vi "בדיקת מפל מתח בין הדקי הממסר תחת עומס 7.vi"(8 "error":errorcluster, 11 "Path for Log":path) -> (0 "error IO":errorcluster, 1 "בטווח כן/לא":bool, 2 "מפל מתח בין דקי הממסר תחת עומס":dbl, 3 "תוצאה זמנית":dbl)   [LabVIEW 2015]
uses:
  M9700 Driver/85/vi.lib/M9700 Modbus.llb/CTL Register Address.ctl
  M9700 Driver/86/vi.lib/M9700 Modbus.llb/CTL CMD Register.ctl
  <vilib>/DAQmx/write.llb/DAQmx Write (Digital Bool 1Line 1Point).vi
  <vilib>/Instr/_visa.llb/VISA Configure Serial Port (Instr).vi
  <vilib>/DAQmx/create/channels.llb/DAQmx Create Channel (DO-Digital Output).vi
  <vilib>/DAQmx/miscellaneous.llb/DAQmx Fill In Error Info.vi
panel:
  out "progress":dbl(slide) min=0.0 max=10.0 scale=0.0..10.0
  in  "stop":bool
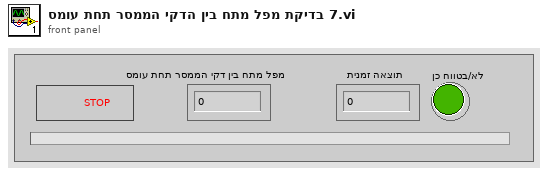
[diagram p1: front panel]
types:
  T1 = enum32{"Invalid", "Standard", "Closed", "Hidden", "Minimized", "Maximized"}
  T2 = typedef "CTL CMD Register.ctl" = u8
  T3 = typedef "CTL Register Address.ctl" = u16
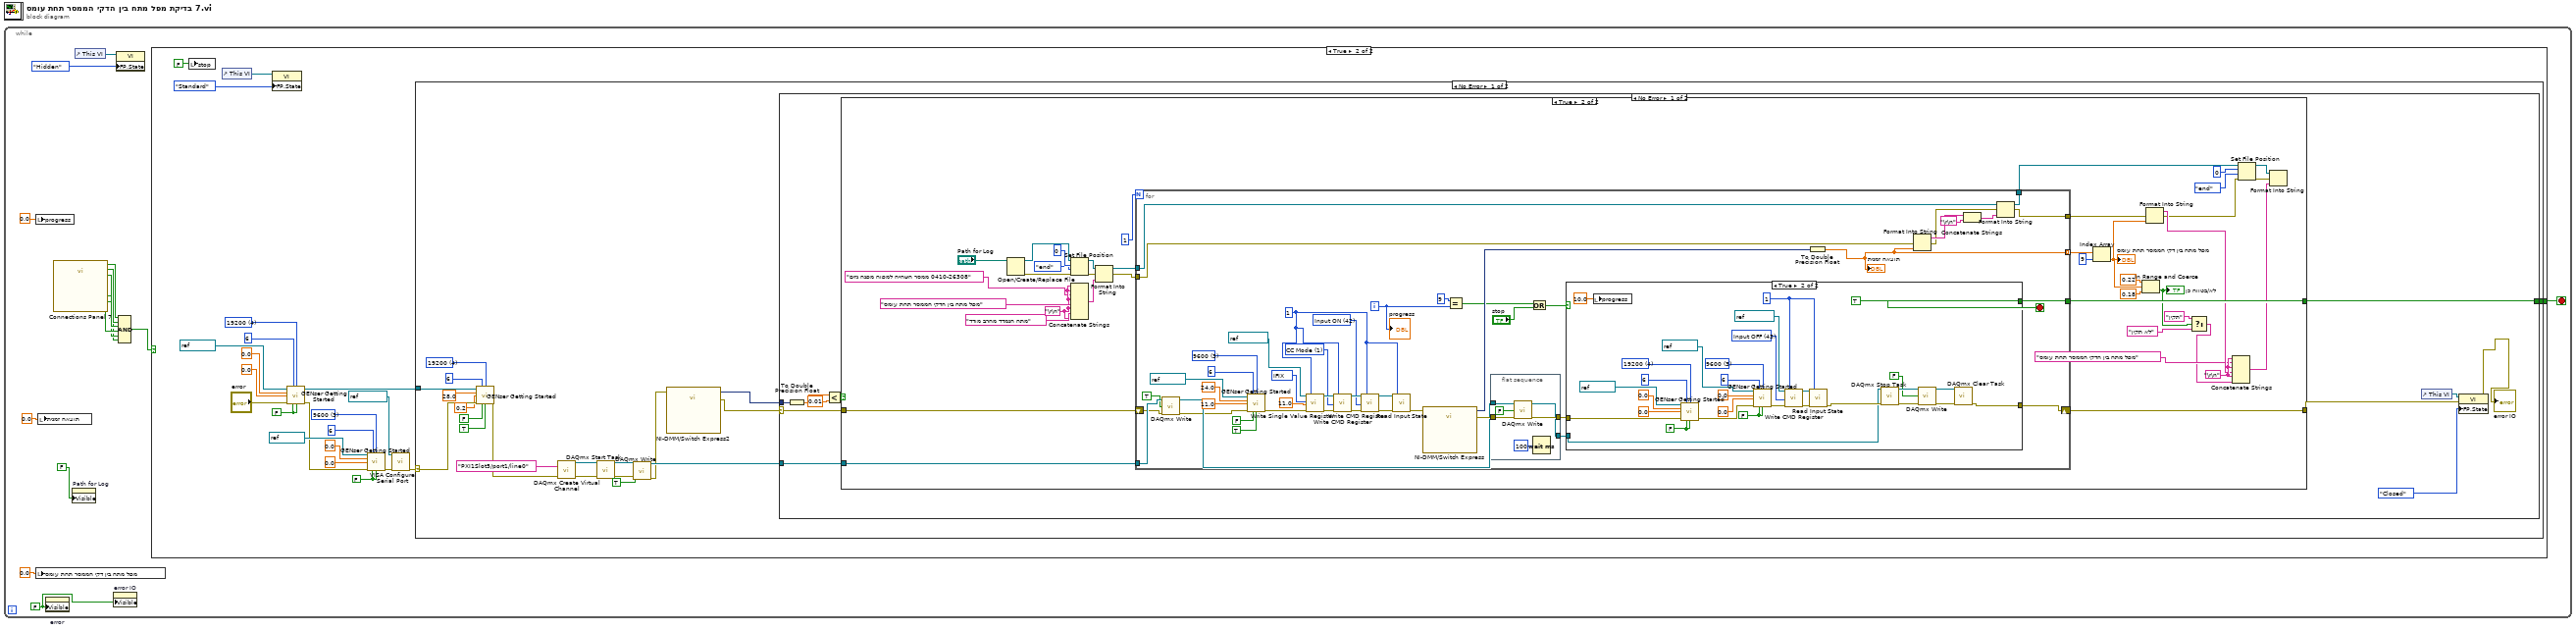
[diagram p0: block diagram]
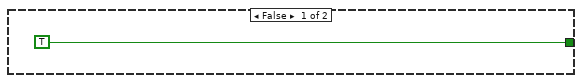
[diagram p2: hidden frame]
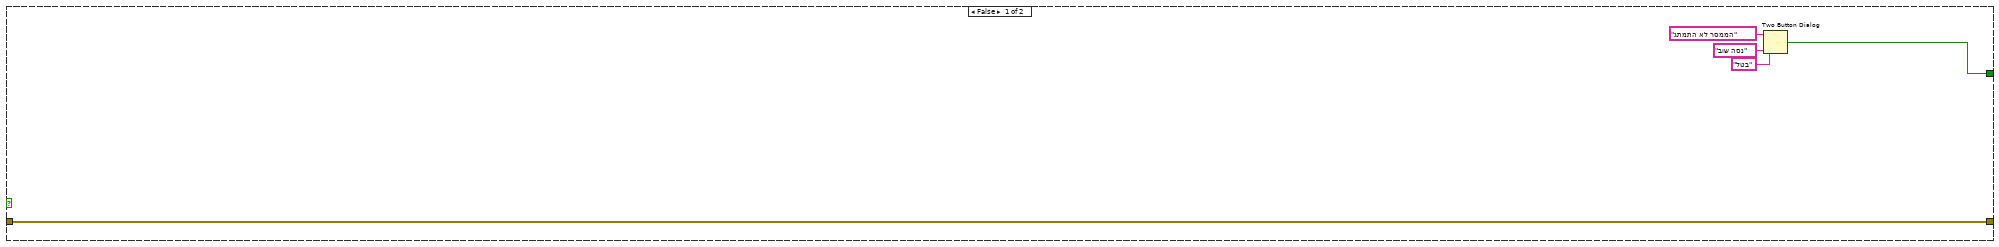
[diagram p3: hidden frame]
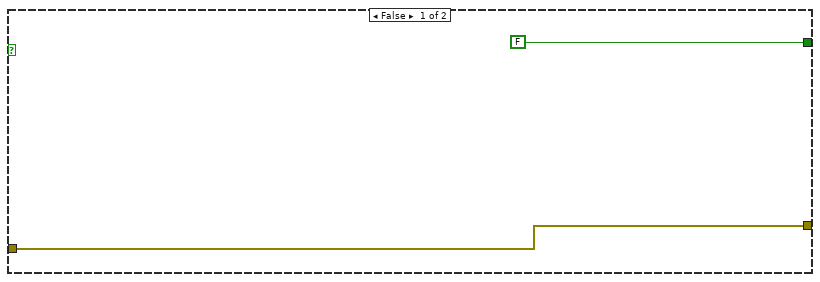
[diagram p4: hidden frame]
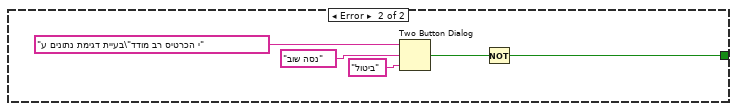
[diagram p5: hidden frame]
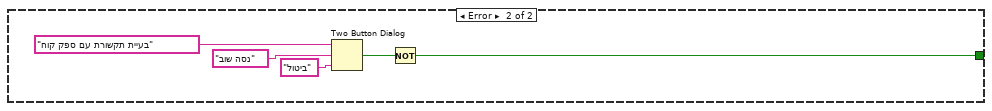
[diagram p6: hidden frame]
diagram:
  n1 = while {
    stop <- w15 stop-if-true
    w9 = FALSE ("Visible")
    n2 = local write "progress"(0.0 ("progress")) -> ()
    n3 = local write "מפל מתח בין דקי הממסר תחת עומס"(0.0 ("מפל מתח בין דקי הממסר תחת עומס")) -> ()
    n4 = local write "תוצאה זמנית"(0.0 ("תוצאה זמנית")) -> ()
    n5 = property on="error" class="Clust (strict)"("Visible"=w9) -> ()  [unwired: 2 in, 2 out]
    n6 = call "Connections Panel 7.vi"() -> ("Input Name 10"=w3:bool, "Input Name 6"=w7:bool, "Input Name 7"=w6:bool, "Input Name 8"=w5:bool, "Input Name 9"=w4:bool, "OK"=w2:bool)  [unwired: 13 in, 1 out]
    n7 = property on="Path for Log" class="Path"("Visible"=FALSE) -> ()  [unwired: 2 in, 2 out]
    n8 = control-ref of="This VI"() -> (w13:refnum<vi>)
    n9 = property on="error IO" class="Clust (strict)"("Visible"=w9) -> ()  [unwired: 2 in, 2 out]
    n10 = property class="VI"(reference=w13, "FP.State"=T1."Hidden" ("Front Panel Window:State")) -> ()  [unwired: 1 in, 2 out]
    n11 = Compound Arithmetic op=AND(w7, w6, w5, w4, w3, w2) -> (w1:bool)
    n12 = case shown="True" w1 {
      tunnel: [TRUE w25] -> w15
      frame False {
      }
      frame True {
        w21 = FALSE ("Reset (T)")
        w30 = u16 3 items=["1200", "2400", "4800", "9600", "19200"] ("BAUD")
        w20 = FALSE ("Output On (T)")
        w35 = u16 4 items=["1200", "2400", "4800", "9600", "19200"] ("BAUD")
        n13 = local write "stop"(FALSE ("stop")) -> ()
        n14 = control-ref of="This VI"() -> (w18:refnum<vi>)
        n15 = property class="VI"(reference=w18, "FP.State"=T1."Standard" ("Front Panel Window:State")) -> ()  [unwired: 1 in, 2 out]
        n16 = call "GENser Getting Started.vi"("VISA"=refnum<visa-resource-name> "COM6", "GEN Addr"=i16 6, "BAUD"=w35, "Voltage Limit"=0.0, "Current Limit"=0.0, "error"="error", "Reset (T)"=w20, "Output On (T)"=w20) -> ("VISA out"=w37:refnum<visa-resource-name>, "error out"=w26:errorcluster)  [unwired: 4 in, 2 out]
        n17 = call "GENser Getting Started.vi"("VISA"=refnum<visa-resource-name> "COM4", "GEN Addr"=i16 6, "BAUD"=w30, "Voltage Limit"=0.0, "Current Limit"=0.0, "error"=w26, "Reset (T)"=w21, "Output On (T)"=w21) -> ("error out"=w23:errorcluster)  [unwired: 4 in, 3 out]
        n18 = call-poly "VISA Configure Serial Port"("VISA resource name"=refnum<visa-resource-name> "COM13", "error in (no error)"=w23) -> ("error out"=w22:errorcluster)  [unwired: 4 in, 9 out]
        n19 = case shown="No Error" w22 {
          selector: w22 -> [w55 _]
          tunnel: w37 -> [w58 _]
          tunnel: [w57 w203] -> w25
          frame No Error {
            w49 = u16 4 items=["1200", "2400", "4800", "9600", "19200"] ("BAUD")
            n20 = call "GENser Getting Started.vi"("VISA"=w58, "GEN Addr"=i16 6, "BAUD"=w49, "Voltage Limit"=28.0, "Current Limit"=0.2, "error"=w55, "Reset (T)"=FALSE, "Output On (T)"=TRUE) -> ("error out"=w44:errorcluster)  [unwired: 4 in, 3 out]
            n21 = call-poly <vilib>:"DAQmx Create Virtual Channel.vi"("lines"=tag "PXI1Slot5/port1/line0", "error in"=w44) -> ("task out"=w47:refnum<k21>, "error out"=w48:errorcluster)  [unwired: 12 in]
            n22 = call <vilib>:"DAQmx Start Task.vi"("task/channels in"=w47, "error in"=w48) -> ("task out"=w43:refnum<k21>, "error out"=w41:errorcluster)  [unwired: 12 in]
            n23 = call-poly <vilib>:"DAQmx Write.vi"("task/channels in"=w43, "data"=TRUE, "error in"=w41) -> ("task out"=w42:refnum<k21>, "error out"=w40:errorcluster)  [unwired: 10 in, 1 out]
            n24 = call "NI-DMM/Switch Express2"("error in"=w40) -> ("signals out"=w56:dynamicdata, "error out"=w45:errorcluster)  [unwired: 16 in, 1 out]
            n25 = case shown="No Error" w45 {
              selector: w45 -> [w67 _]
              tunnel: [w66 w198] -> w57
              tunnel: w56 -> [w69 _]
              tunnel: w42 -> [w60 _]
              frame No Error {
                n26 = To Double Precision Float(number=w69) -> (double precision float=w65:dbl)
                n27 = Less?(x=w65, y=0.01) -> (x < y?=w68:bool)
                n28 = case shown="True" w68 {
                  tunnel: w67 -> [w74 w111]
                  tunnel: [w70 w112] -> w66
                  tunnel: [w74 w105] -> w61
                  tunnel: w60 -> [_ w106]
                  frame False {
                    n29 = Two Button Dialog(message="הממסר לא התמתג", 1:"נסה שוב" ("F button name (\"Cancel\")"), 2:"בטל" ("T button name (\"OK\")")) -> (T button?=w70:bool)
                  }
                  frame True {
                    w91 = "\r\n"
                    w94 = "\r\n"
                    n30 = Open/Create/Replace File(file path (use dialog)="Path for Log") -> (refnum out=w102:refnum<file>, error out=w101:errorcluster)  [unwired: 5 in, 1 out]
                    n31 = Set File Position(offset (in bytes) (0)=i64 0, refnum=w102, from (0:start)=enum16{"start", "end", "current"}."end", error in=w101) -> (refnum out=w98:refnum<file>, error out=w95:errorcluster)
                    n32 = Concatenate Strings(w94, w94, "ממסר השהייה למפוח מפנה גזים 0410-26308", w94, "מפל מתח בין הדקי הממסר תחת עומס", w94, "מתח הנמדד מהרב מודד", w94) -> (w100:string)
                    n33 = Format Into String(initial string=w98, error in=w95, w100) -> (resulting string=w92:refnum<file>, error out=w93:errorcluster)  [unwired: 1 in]
                    n34 = for {
                      N: 1 -> [_]
                      tunnel: [w135] -> w112
                      shift-right: [w132] -> w105
                      shift-left: w111 -> [w127]
                      tunnel: [w114] -> w110 mode=indexing
                      tunnel: w106 -> [w128]
                      tunnel: w93 -> [w117]
                      tunnel: w92 -> [w119]
                      tunnel: [w116] -> w85
                      tunnel: [w115] -> w76
                      i -> [w131]
                      stop <- w135 stop-if-true
                      w143 = T2 42 items=["CC Mode"=1, "CV Mode"=2, "CW Mode"=3, "CR Mode"=4, "Short Mode"=26, "Set SysPara"=41, "Input ON"=42, "Input OFF"=43] ("CMD Register Value")
                      w146 = u8 1 ("Load Address")
                      w150 = T2 1 items=["CC Mode"=1, "CV Mode"=2, "CW Mode"=3, "CR Mode"=4, "Short Mode"=26, "Set SysPara"=41, "Input ON"=42, "Input OFF"=43] ("CMD Register Value")
                      w153 = T3 2561 items=["REMOTE"=1283, "ISTATE"=1296, "CMD"=2560, "IFIX"=2561, "UFIX"=2563, "PFIX"=2565, "RFIX"=2567, "IMAX"=2612, "UMAX"=2614, "PMAX"=2616, "U"=2816, "I"=2818, "MODEL"=2822, "EDITION"=2823] ("Register Address")
                      w158 = u16 3 items=["1200", "2400", "4800", "9600", "19200"] ("BAUD")
                      n35 = call-poly <vilib>:"DAQmx Write.vi"("task/channels in"=w128, "data"=TRUE, "error in"=w127) -> ("task out"=w126:refnum<k21>, "error out"=w125:errorcluster)  [unwired: 10 in, 1 out]
                      n36 = call "GENser Getting Started.vi"("VISA"=refnum<visa-resource-name> "COM4", "GEN Addr"=i16 6, "BAUD"=w158, "Voltage Limit"=24.0, "Current Limit"=11.0, "error"=w125, "Reset (T)"=FALSE, "Output On (T)"=TRUE) -> ("error out"=w148:errorcluster)  [unwired: 4 in, 3 out]
                      n37 = call "Write Single Value Register.vi"("VISA resource name"=refnum<visa-resource-name> "COM13", "Starting Address(HEX)"=w153, "Register Single Value"=sgl 11.0, "error in"=w148, "Load Address"=w146) -> ("VISA resource name out"=w152:refnum<visa-resource-name>, "error out"=w151:errorcluster)  [unwired: 13 out]
                      n38 = call "Write CMD Register.vi"("VISA resource name"=w152, "CMD Value"=w150, "error in"=w151, "Load Address"=w146) -> ("VISA resource name out"=w147:refnum<visa-resource-name>, "error out"=w144:errorcluster)  [unwired: 14 out]
                      n39 = call "Write CMD Register.vi"("VISA resource name"=w147, "CMD Value"=w143, "error in"=w144, "Load Address"=w146) -> ("VISA resource name out"=w145:refnum<visa-resource-name>, "error out"=w142:errorcluster)  [unwired: 14 out]
                      n40 = call "Read Input State.vi"("VISA resource name"=w145, "error in"=w142, "Load Address"=w146) -> ("error out"=w141:errorcluster)  [unwired: 16 out]
                      n41 = call "NI-DMM/Switch Express"("error in"=w141) -> ("signals out"=w140:dynamicdata, "error out"=w129:errorcluster)  [unwired: 16 in, 1 out]
                      n42 = Equal?(x=9, y=w131) -> (x = y?=w137:bool)
                      n43 = flat-sequence {
                        tunnel: [w165] -> w130
                        tunnel: w129 -> [w164]
                        tunnel: w126 -> [w162]
                        tunnel: [w161] -> w123
                        frame #0 {
                          n44 = call-poly <vilib>:"DAQmx Write.vi"("task/channels in"=w162, "data"=FALSE, "error in"=w164) -> ("task out"=w161:refnum<k21>, "error out"=w165:errorcluster)  [unwired: 10 in, 1 out]
                          n45 = Wait (ms)(milliseconds to wait=u32 100) -> ()  [unwired: 1 out]
                        }
                      }
                      n46 = Or(x=w137, y="stop") -> (x .or. y?=w138:bool)
                      n47 = case shown="True" w138 {
                        tunnel: [FALSE TRUE] -> w135
                        tunnel: w130 -> [w166 w186]
                        tunnel: [w166 w169] -> w132
                        tunnel: w123 -> [_ w168]
                        frame False {
                        }
                        frame True {
                          w177 = u8 1 ("Load Address")
                          w180 = T2 43 items=["CC Mode"=1, "CV Mode"=2, "CW Mode"=3, "CR Mode"=4, "Short Mode"=26, "Set SysPara"=41, "Input ON"=42, "Input OFF"=43] ("CMD Register Value")
                          w184 = FALSE ("Reset (T)")
                          w190 = u16 3 items=["1200", "2400", "4800", "9600", "19200"] ("BAUD")
                          w183 = FALSE ("Reset (T)")
                          w193 = u16 4 items=["1200", "2400", "4800", "9600", "19200"] ("BAUD")
                          n48 = local write "progress"(10.0 ("progress")) -> ()
                          n49 = call "GENser Getting Started.vi"("VISA"=refnum<visa-resource-name> "COM6", "GEN Addr"=i16 6, "BAUD"=w193, "Voltage Limit"=0.0, "Current Limit"=0.0, "error"=w186, "Reset (T)"=w183, "Output On (T)"=w183) -> ("error out"=w185:errorcluster)  [unwired: 4 in, 3 out]
                          n50 = call "GENser Getting Started.vi"("VISA"=refnum<visa-resource-name> "COM4", "GEN Addr"=i16 6, "BAUD"=w190, "Voltage Limit"=0.0, "Current Limit"=0.0, "error"=w185, "Reset (T)"=w184, "Output On (T)"=w184) -> ("error out"=w182:errorcluster)  [unwired: 4 in, 3 out]
                          n51 = call "Write CMD Register.vi"("VISA resource name"=refnum<visa-resource-name> "COM13", "CMD Value"=w180, "error in"=w182, "Load Address"=w177) -> ("VISA resource name out"=w178:refnum<visa-resource-name>, "error out"=w181:errorcluster)  [unwired: 14 out]
                          n52 = call "Read Input State.vi"("VISA resource name"=w178, "error in"=w181, "Load Address"=w177) -> ("error out"=w170:errorcluster)  [unwired: 16 out]
                          n53 = call <vilib>:"DAQmx Stop Task.vi"("task/channels in"=w168, "error in"=w170) -> ("task out"=w175:refnum<k21>, "error out"=w173:errorcluster)  [unwired: 12 in]
                          n54 = call-poly <vilib>:"DAQmx Write.vi"("task/channels in"=w175, "data"=FALSE, "error in"=w173) -> ("task out"=w172:refnum<k21>, "error out"=w171:errorcluster)  [unwired: 10 in, 1 out]
                          n55 = call <vilib>:"DAQmx Clear Task.vi"("task in"=w172, "error in"=w171) -> ("error out"=w169:errorcluster)  [unwired: 13 in]
                        }
                      }
                      n56 = To Double Precision Float(number=w140) -> (double precision float=w114:dbl)
                      "תוצאה זמנית" <- w114
                      n57 = Format Into String(error in=w117, w114) -> (resulting string=w121:string, error out=w118:errorcluster)  [unwired: 2 in]
                      n58 = Concatenate Strings(w121, "\r\n") -> (w120:string)
                      n59 = Format Into String(initial string=w119, error in=w118, w120) -> (resulting string=w116:refnum<file>, error out=w115:errorcluster)  [unwired: 1 in]
                      "progress" <- w131
                    }
                    n60 = Index Array(array=w110, index=9) -> (element=w84:dbl)
                    "מפל מתח בין דקי הממסר תחת עומס" <- w84
                    n61 = In Range and Coerce(upper limit=0.22, x=w84, lower limit=0.18) -> (In Range?=w79:bool)  [unwired: 1 out]
                    "בטווח כן/לא" <- w79
                    n62 = Format Into String(error in=w76, w84) -> (resulting string=w83:string, error out=w77:errorcluster)  [unwired: 2 in]
                    n63 = Select(t="תקין", s=w79, f="לא תקין") -> (s? t:f=w78:string)
                    n64 = Concatenate Strings(w91, "מפל מתח בין הדקי הממסר תחת עומס" ("string"), w91, w83, w91, w78) -> (w86:string)
                    n65 = Set File Position(offset (in bytes) (0)=i64 0, refnum=w85, from (0:start)=enum16{"start", "end", "current"}."end", error in=w77) -> (refnum out=w88:refnum<file>, error out=w87:errorcluster)
                    n66 = Format Into String(initial string=w88, error in=w87, w86) -> ()  [unwired: 1 in, 2 out]
                  }
                }
                n67 = control-ref of="This VI"() -> (w63:refnum<vi>)
                n68 = property class="VI"(reference=w63, error in=w61, "FP.State"=T1."Closed" ("Front Panel Window:State")) -> (error out=→"error IO":errorcluster)  [unwired: 1 out]
              }
              frame Error {
                n69 = Two Button Dialog(message="בעיית דגימת נתונים ע\"י הכרטיס רב מודד", 1:"ביטול" ("F button name (\"Cancel\")"), 2:"נסה שוב" ("T button name (\"OK\")")) -> (T button?=w199:bool)
                n70 = Not(x=w199) -> (.not. x?=w198:bool)
              }
            }
          }
          frame Error {
            n71 = Two Button Dialog(message="בעיית תקשורת עם ספק קוח", 1:"ביטול" ("F button name (\"Cancel\")"), 2:"נסה שוב" ("T button name (\"OK\")")) -> (T button?=w204:bool)
            n72 = Not(x=w204) -> (.not. x?=w203:bool)
          }
        }
      }
    }
  }
